vi "quaternion.vi"(9 "error in (no error)":errorcluster, 10 "COM Bluegiga in":refnum<visa-resource-name>) -> (0 "Z_Q":ext, 1 "Y_Q":ext, 2 "X_Q":ext, 3 "W_Q":ext, 5 "COM Bluegiga out":refnum<visa-resource-name>, 7 "error out":errorcluster)   [LabVIEW 2020]
panel:
  out "characteristic value":u8[](array[numeric])
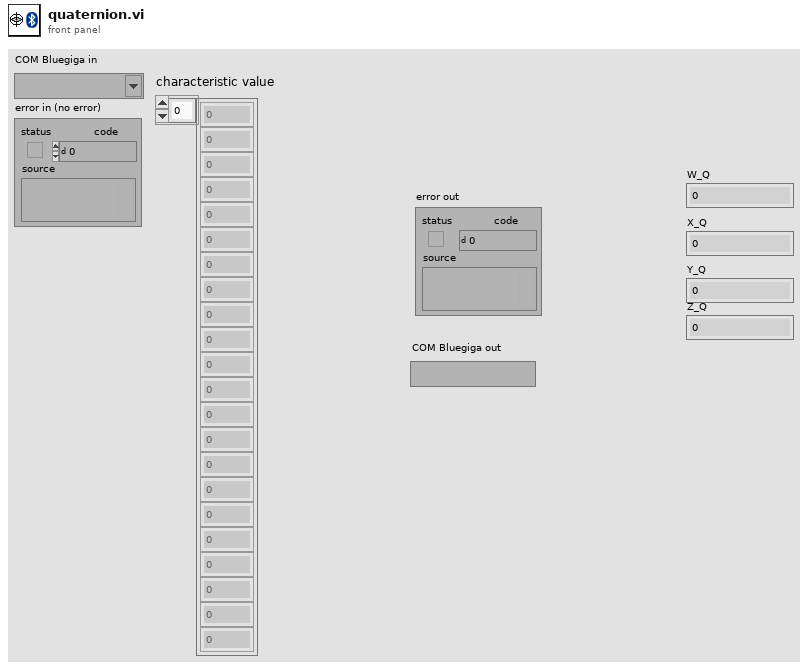
[diagram p1: front panel]
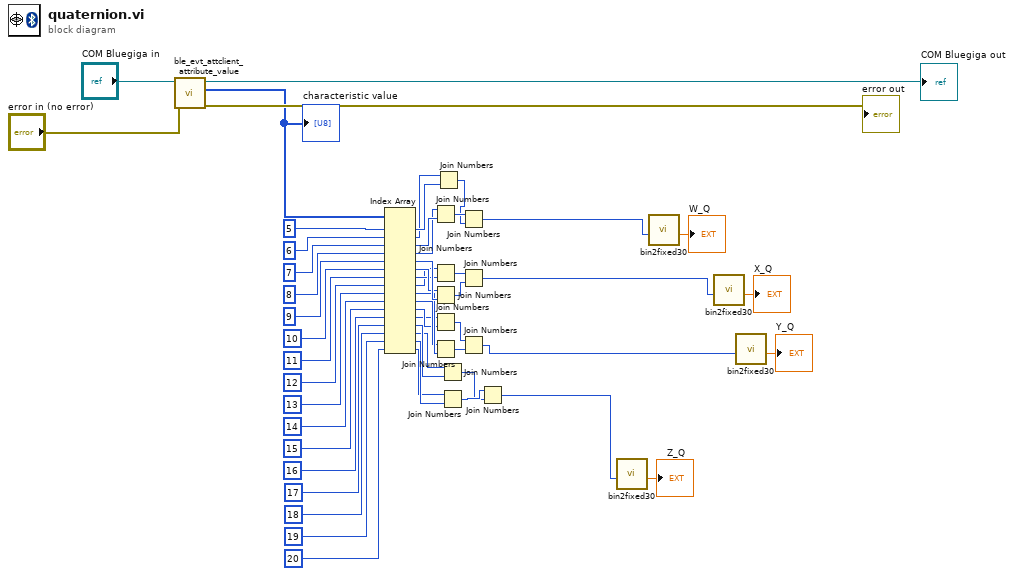
[diagram p0: block diagram]
diagram:
  n1 = call <vilib>:"ble_evt_attclient_attribute_value.vi"("error in (no error)"="error in (no error)", "COM Bluegiga in"="COM Bluegiga in") -> ("error out"=→"error out":errorcluster, "characteristic value"=w19:u8[], "COM Bluegiga out"=→"COM Bluegiga out":refnum<visa-resource-name>)  [unwired: 6 in, 1 out]
  "characteristic value" <- w19
  n2 = Index Array(array=w19, index #1=5 ("index"), index #2=6 ("index"), index #3=7 ("index"), index #4=8 ("index"), index #5=9 ("index"), index #6=10 ("index"), index #7=11 ("index"), index #8=12 ("index"), index #9=13 ("index"), index #10=14 ("index"), index #11=15 ("index"), index #12=16 ("index"), index #13=17 ("index"), index #14=18 ("index"), index #15=19 ("index"), index #16=20 ("index")) -> (element #1=w37:u8, element #2=w36:u8, element #3=w35:u8, element #4=w34:u8, element #5=w33:u8, element #6=w32:u8, element #7=w31:u8, element #8=w30:u8, element #9=w27:u8, element #10=w26:u8, element #11=w25:u8, element #12=w24:u8, element #13=w14:u8, element #14=w13:u8, element #15=w12:u8, element #16=w11:u8)
  n3 = Join Numbers(hi=w34, lo=w35) -> ((hi.lo)=w21:u16)
  n4 = Join Numbers(hi=w30, lo=w31) -> ((hi.lo)=w28:u16)
  n5 = Join Numbers(hi=w32, lo=w33) -> ((hi.lo)=w29:u16)
  n6 = Join Numbers(hi=w24, lo=w25) -> ((hi.lo)=w22:u16)
  n7 = Join Numbers(hi=w26, lo=w27) -> ((hi.lo)=w23:u16)
  n8 = Join Numbers(hi=w36, lo=w37) -> ((hi.lo)=w20:u16)
  n9 = Join Numbers(hi=w13, lo=w14) -> ((hi.lo)=w8:u16)
  n10 = Join Numbers(hi=w11, lo=w12) -> ((hi.lo)=w9:u16)
  n11 = Join Numbers(hi=w21, lo=w20) -> ((hi.lo)=w4:u32)
  n12 = Join Numbers(hi=w28, lo=w29) -> ((hi.lo)=w3:u32)
  n13 = Join Numbers(hi=w22, lo=w23) -> ((hi.lo)=w2:u32)
  n14 = Join Numbers(hi=w9, lo=w8) -> ((hi.lo)=w1:u32)
  n15 = call "bin2fixed30.vi"("number"=w1) -> ("Result"=→"Z_Q":ext)  [unwired: 10 in]
  n16 = call "bin2fixed30.vi"("number"=w4) -> ("Result"=→"W_Q":ext)  [unwired: 10 in]
  n17 = call "bin2fixed30.vi"("number"=w3) -> ("Result"=→"X_Q":ext)  [unwired: 10 in]
  n18 = call "bin2fixed30.vi"("number"=w2) -> ("Result"=→"Y_Q":ext)  [unwired: 10 in]
